vi "PKG_IMC_PWMpropFollow.vi"(0 "handle":u32, 1 "PWMend":dbl, 2 "ch":i32, 3 "axis":i32, 5 "polar":i32, 7 "freq":dbl, 9 "PWMstart":dbl, 10 "paramEnd":i32, 12 "offset":dbl, 13 "paramloc":i32, 14 "paramStart":i32) -> (4 "handle out":u32, 6 "function return":i32)   [LabVIEW 2011, in "IMC_Pkg4xxx.lvlib"]
doc: "PKG_IMC_PWMpropFollow(IMC_HANDLE handle, int polar, double freq, double PWMstart, double PWMend, double offset, int ch, int paramloc, int axis, int paramStart, int paramEnd);"
uses:
  IMC_Pkg4xxx.lvlib
  IMC_Pkg4xxx.dll
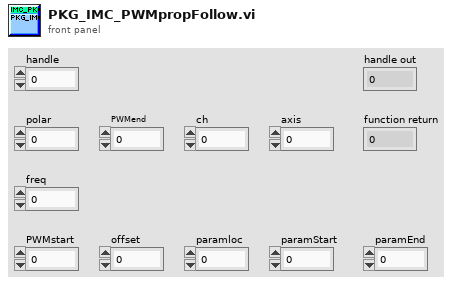
[diagram p1: front panel]
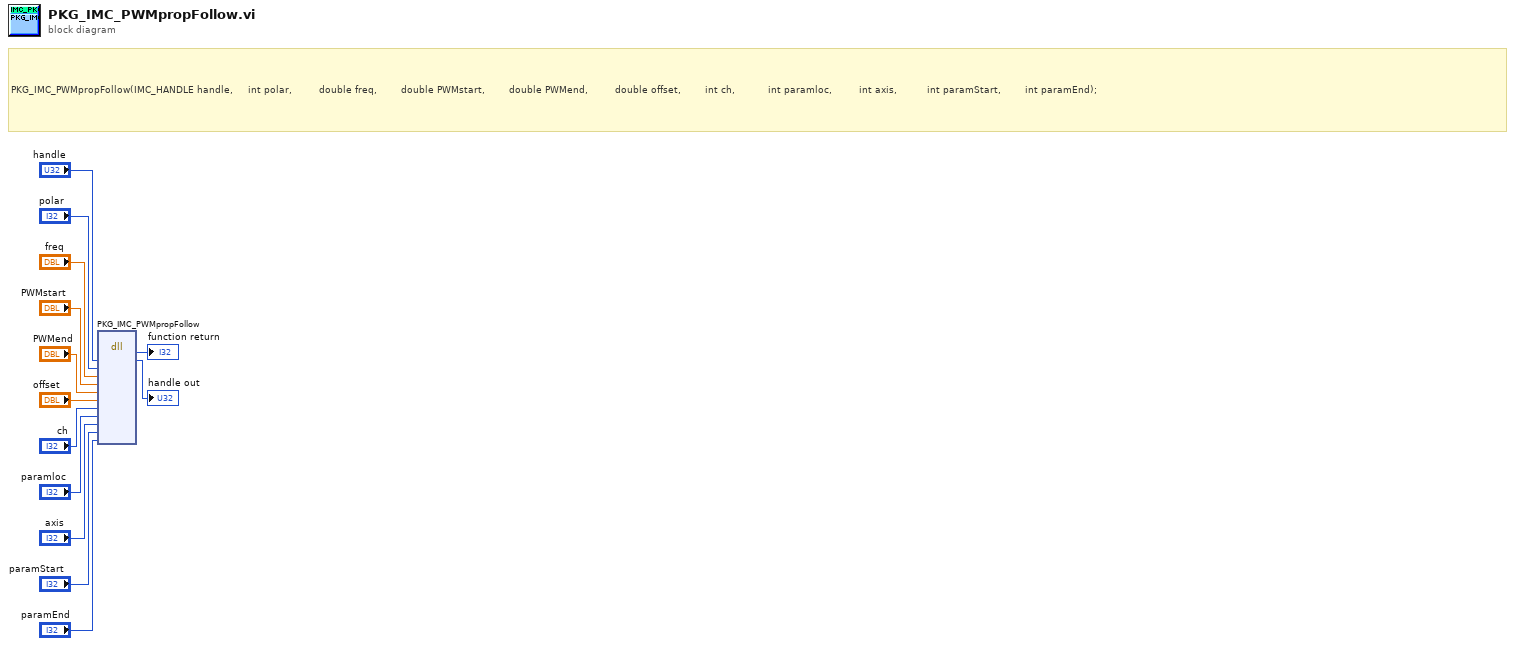
[diagram p0: block diagram]
diagram:
  # "PKG_IMC_PWMpropFollow(IMC_HANDLE handle,\t\t\t\t\tint polar,\t\t\t\t\t\t\t\t\tdouble freq,\t\t\t\t\t\t\t\tdouble PWMstart, \t\t\t\t\t\t\tdouble PWMend, \t\t\t\t\t\t\t\tdouble offset,\t\t\t\t\t\t\t\tint ch,\t\t\t\t\t\t \t\t\t\tint paramloc, \t\t\t\t\t\t\t\tint axis, \t\t\t\t\t\t\t\t\tint paramStart, \t\t\t\t\t\t\tint paramEnd);"
  n1 = dll-call lib="PTH1mabs F光盘刻录\niMC MotionIMCNet_V4.0IMCAppincLabviewIMC_PKG4xxxIMC_PKG4xxx\nIMC_Pkg4xxx.*" fn="PKG_IMC_PWMpropFollow"("handle"="handle", "polar"="polar", "freq"="freq", "PWMstart"="PWMstart", "PWMend"="PWMend", "offset"="offset", "ch"="ch", "paramloc"="paramloc", "axis"="axis", "paramStart"="paramStart", "paramEnd"="paramEnd") -> (→"function return":i32, "handle"=→"handle out":u32)  [unwired: 13 in, 2 out]
